vi "Write applicationHandler.vi"(10 "ApplicationHandler.lvclass":refnum<class "ApplicationHandler.lvclass">, 11 "ComponentData in":refnum<class "ComponentData.lvclass">) -> (3 "ComponentData out":refnum<class "ComponentData.lvclass">)   [LabVIEW 2013, in "ComponentData.lvlib" / "ComponentData.lvclass"]
uses:
  <userlib>/Common/Component/common_application/RT/ComponentData/ComponentData/ComponentData.lvclass
  <userlib>/Common/Component/common_application/RT/ComponentData/ApplicationHandler/ApplicationHandler.lvclass
  <userlib>/Common/Component/common_application/RT/ComponentData/ComponentData/ComponentData.lvclass/ComponentData.ctl
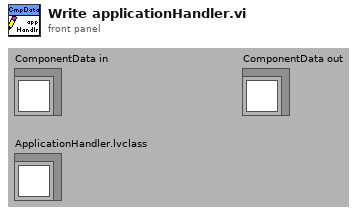
[diagram p1: front panel]
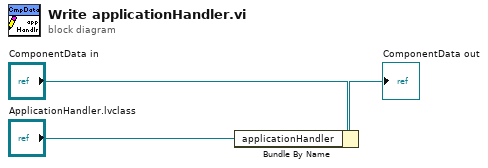
[diagram p0: block diagram]
diagram:
  n1 = Bundle By Name(cluster="ComponentData in", "applicationHandler"="ApplicationHandler.lvclass") -> (→"ComponentData out":refnum<class "ComponentData.lvclass">)
